vi "Andor_iXon_Init_Point-Picture.vi"(8 "Input Cluster 2":T6, 11 "Cluster":T7) -> (0 "Output Cluster":T6)   [LabVIEW 2009]
uses:
  atmcd32d.llb/AcquisitionMode_mode typedef.ctl
  atmcd32d.llb/ReadMode_mode typedef.ctl
  atmcd32d.llb/TriggerMode_mode typedef.ctl
  atmcd32d.llb/Shutter_type typedef.ctl
  atmcd32d.llb/Shutter_mode typedef.ctl
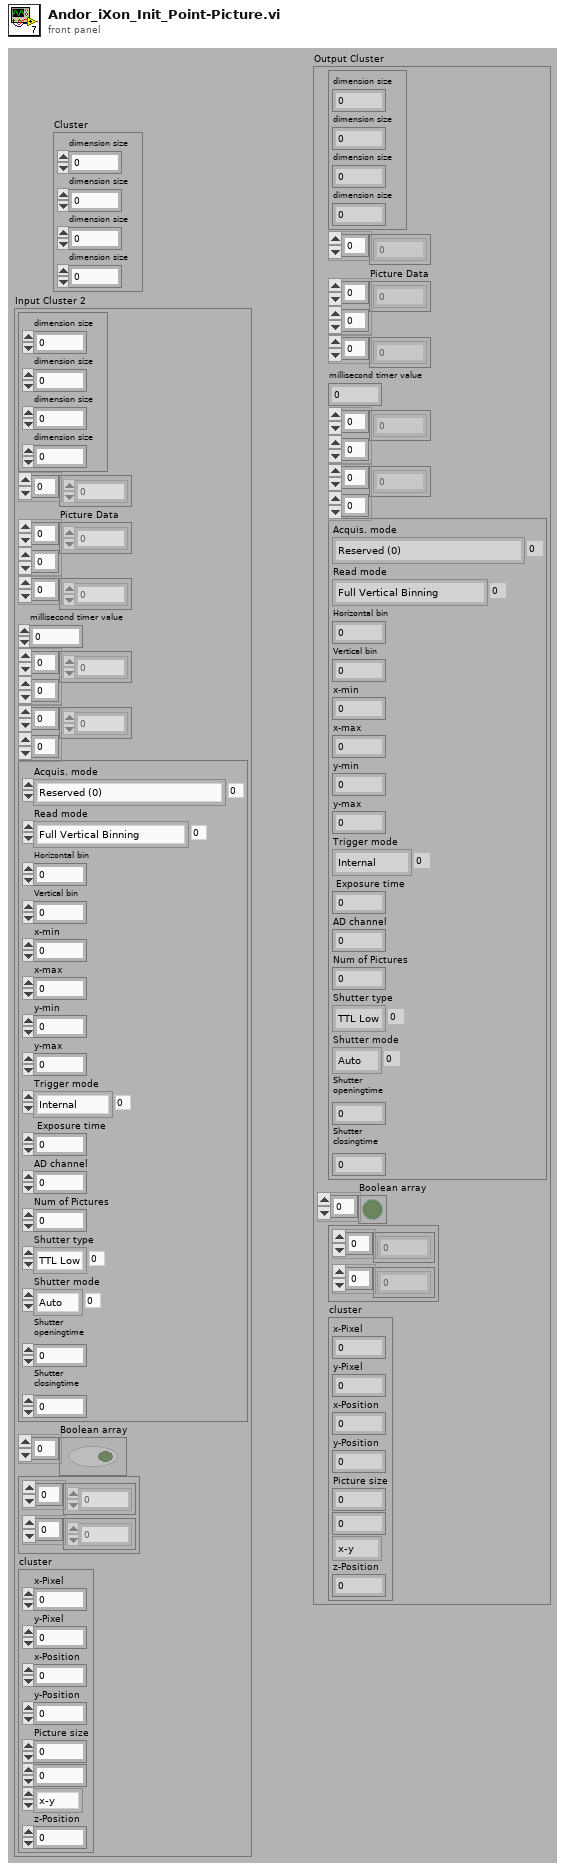
[diagram p1: front panel]
types:
  T1 = typedef "AcquisitionMode_mode typedef.ctl" = enum16{"Reserved (0)", "Single Scan", "Accumulate", "Kinetics", "Fast Kinetics", "Run Till Abort", "Reserved (6)", "Reserved (7)", "Reserved (8)", "Time Delayed Integration"}
  T2 = typedef "ReadMode_mode typedef.ctl" = enum16{"Full Vertical Binning", "Multi-Track", "Random-Track", "Single-Track", "Image"}
  T3 = typedef "TriggerMode_mode typedef.ctl" = enum16{"Internal", "External", "N/A (2)", "N/A (3)", "N/A (4)", "N/A (5)", "External Start"}
  T4 = typedef "Shutter_type typedef.ctl" = enum16{"TTL Low", "TTL High"}
  T5 = typedef "Shutter_mode typedef.ctl" = enum16{"Auto", "Open", "Close"}
  T6 = cluster{cluster{"dimension size":i32, "dimension size":i32, "dimension size":i32, "dimension size":i32}, i32[], "Picture Data":dbl[][], u32[], "millisecond timer value":u32, dbl[][], i32[][], cluster{"Acquis. mode":T1, "Read mode":T2, "Horizontal bin":i32, "Vertical bin":i32, "x-min":i32, "x-max":i32, "y-min":i32, "y-max":i32, "Trigger mode":T3, " Exposure time":sgl, "AD channel":i32, "Num of Pictures":i32, "Shutter type":T4, "Shutter mode":T5, "Shutter\nopeningtime":i32, "Shutter\nclosingtime":i32}, "Boolean array":bool[], cluster{dbl[], dbl[]}, "cluster":cluster{"x-Pixel":u16, "y-Pixel":u16, "x-Position":dbl, "y-Position":dbl, "Picture size":dbl, dbl, enum32{"x-y", "x-z", "y-z"}, "z-Position":dbl}}
  T7 = cluster{"dimension size":i32, "dimension size":i32, "dimension size":i32, "dimension size":i32}
  T8 = cluster{"Acquis. mode":T1, "Read mode":T2, "Horizontal bin":i32, "Vertical bin":i32, "x-min":i32, "x-max":i32, "y-min":i32, "y-max":i32, "Trigger mode":T3, " Exposure time":sgl, "AD channel":i32, "Num of Pictures":i32, "Shutter type":T4, "Shutter mode":T5, "Shutter\nopeningtime":i32, "Shutter\nclosingtime":i32}
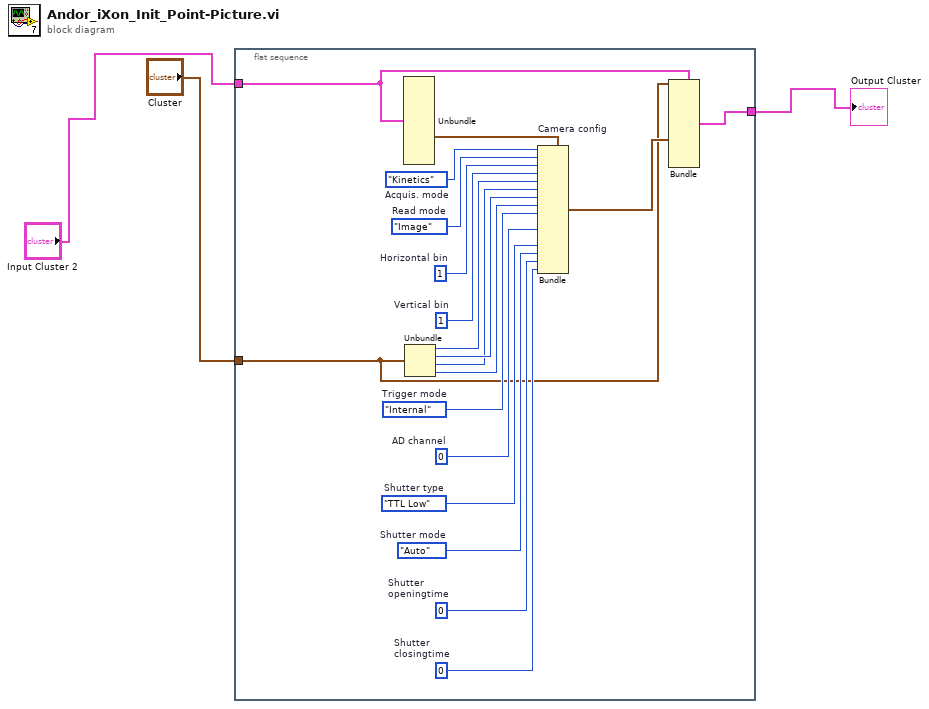
[diagram p0: block diagram]
diagram:
  n1 = flat-sequence {
    tunnel: "Input Cluster 2" -> [w5]
    tunnel: [w8] -> w2
    tunnel: "Cluster" -> [w6]
    frame #0 {
      w16 = 1  # Vertical bin
      w15 = 1  # Horizontal bin
      w22 = 0  # Shutter closingtime
      w21 = 0  # Shutter openingtime
      w20 = Shutter_mode_typedef."Auto"  # Shutter mode
      w19 = Shutter_type_typedef."TTL Low"  # Shutter type
      w18 = 0  # AD channel
      w17 = TriggerMode_mode_typedef."Internal"  # Trigger mode
      w14 = ReadMode_mode_typedef."Image"  # Read mode
      w13 = AcquisitionMode_mode_typedef."Kinetics"  # Acquis. mode
      n2 = Unbundle(w5) -> (w4:T8)  [unwired: 10 out]
      n3 = Unbundle(w6) -> ("dimension size"=w12:i32, "dimension size"=w11:i32, "dimension size"=w10:i32, "dimension size"=w9:i32)
      n4 = Bundle "Camera config"(cluster=w4, "Acquis. mode"=w13, "Read mode"=w14, "Horizontal bin"=w15, "Vertical bin"=w16, "x-min"=w12, "x-max"=w10, "y-min"=w11, "y-max"=w9, "Trigger mode"=w17, "AD channel"=w18, "Shutter type"=w19, "Shutter mode"=w20, "Shutter\nopeningtime"=w21, "Shutter\nclosingtime"=w22) -> (w7:T8)  [unwired: 2 out]
      n5 = Bundle(cluster=w5, w6, w7) -> (w8:T6)  [unwired: 9 out]
    }
  }
  "Output Cluster" <- w2
